vi "ELOG_Control_GetState.vi"(8 "error in (no error)":errorcluster, 11 "OXY_SCPI Reseource In":refnum<visa-resource-name>) -> (0 "error out":errorcluster, 1 "communication_data":T1, 2 "State":string, 3 "OXY_SCPI Reseource Out":refnum<visa-resource-name>)   [LabVIEW 2018, in "OXYGEN.lvlib"]
doc: "Returns the internal state of the ELOG subsystem. This command is not needed for regular operations but is useful for information purposes.\nPossible states are: CONFIG, RUNNING and INVALID"
uses:
  OXYGEN.lvlib
  TypeDefs/Cluster_RawCommData.ctl
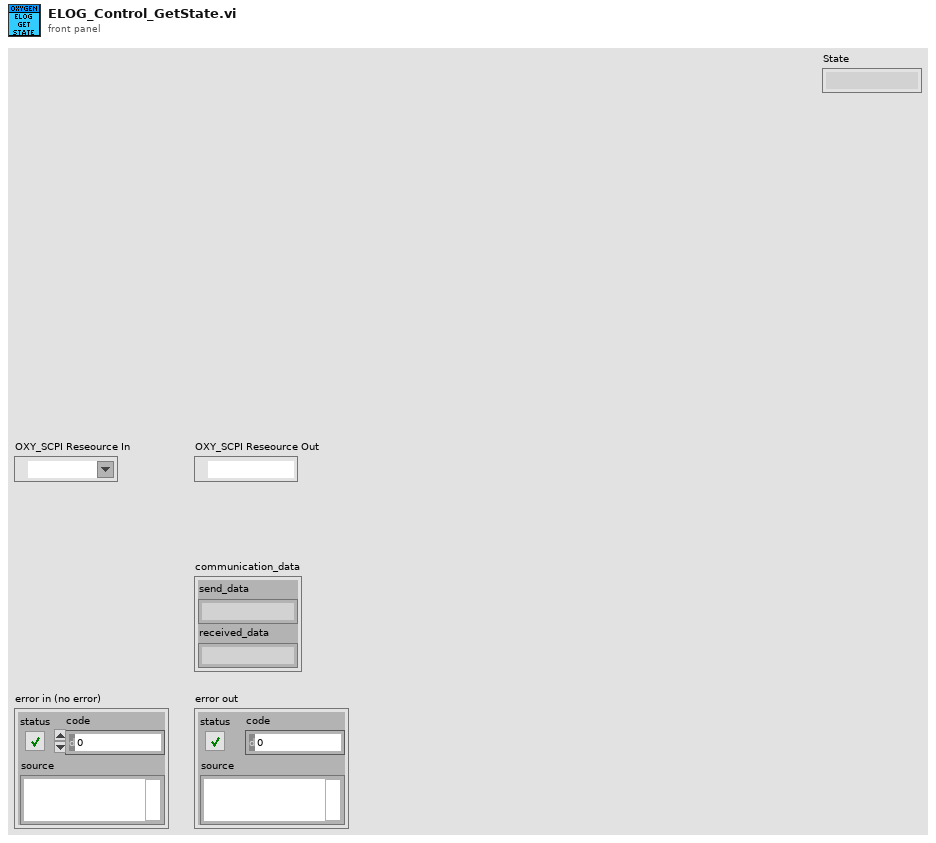
[diagram p1: front panel]
types:
  T1 = typedef "OXYGEN.lvlib/Cluster_RawCommData.ctl" = cluster{"send_data":string, "received_data":string}
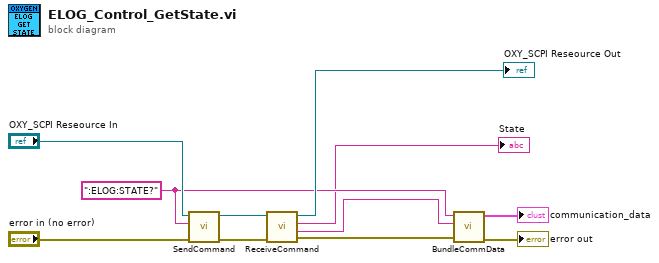
[diagram p0: block diagram]
diagram:
  w3 = ":ELOG:STATE?" ("String to Send")
  n1 = call "SendCommand.vi"("error in (no error)"="error in (no error)", "String to Send"=w3, "OXY_SCPI Reseource In"="OXY_SCPI Reseource In") -> ("error out"=w11:errorcluster, "OXY_SCPI Reseource Out"=w10:refnum<visa-resource-name>)  [unwired: 7 in]
  n2 = call "ReceiveCommand.vi"("error in (no error)"=w11, "OXY_SCPI Reseource In"=w10) -> ("error out"=w2:errorcluster, "received Data with Header"=w4:string, "received Data"=→"State":string, "OXY_SCPI Reseource Out"=→"OXY_SCPI Reseource Out":refnum<visa-resource-name>)  [unwired: 6 in]
  n3 = call "BundleCommData.vi"("error in (no error)"=w2, "received_data"=w4, "send_data"=w3) -> ("error out"=→"error out":errorcluster, "communication_data"=→"communication_data":T1)  [unwired: 7 in]
